vi "計算機.vi"() -> ()   [LabVIEW 2021]
uses:
  <vilib>/gmath/NI_Gmath.lvlib
  <vilib>/regexp/Match Regular Expression.xnode
panel:
  out "113550059":string
  in  "+/-":bool
  in  "1/x":bool
  in  "stop":bool
  out "String 2":string
  in  "pi":bool
  in  "tan":bool
  in  "cos":bool
  in  "sin":bool
  in  "√":bool
  out "String":string
  out "concatenated string":string
  in  "%":bool
  in  "Del":bool
  in  "=":bool
  in  "CE":bool
  in  ")":bool
  in  "(":bool
  out "Answer":string
  in  "1":bool
  in  "/":bool
  in  ".":bool
  in  "0":bool
  in  "*":bool
  in  "3":bool
  in  "2":bool
  in  "-":bool
  in  "6":bool
  in  "5":bool
  in  "4":bool
  in  "+":bool
  in  "9":bool
  in  "8":bool
  in  "7":bool
  # "記錄一"
  # "記錄二"
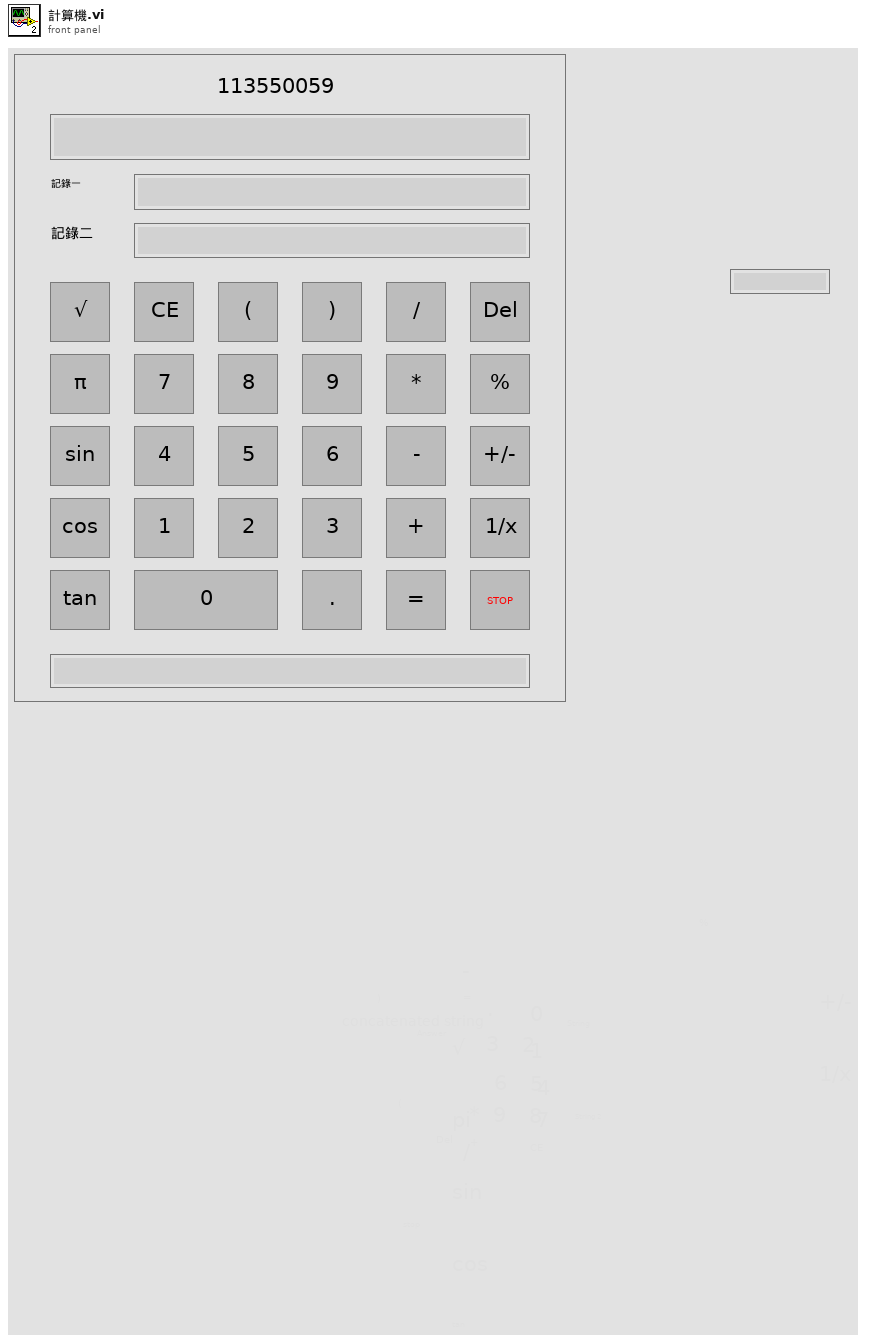
[diagram p1: front panel]
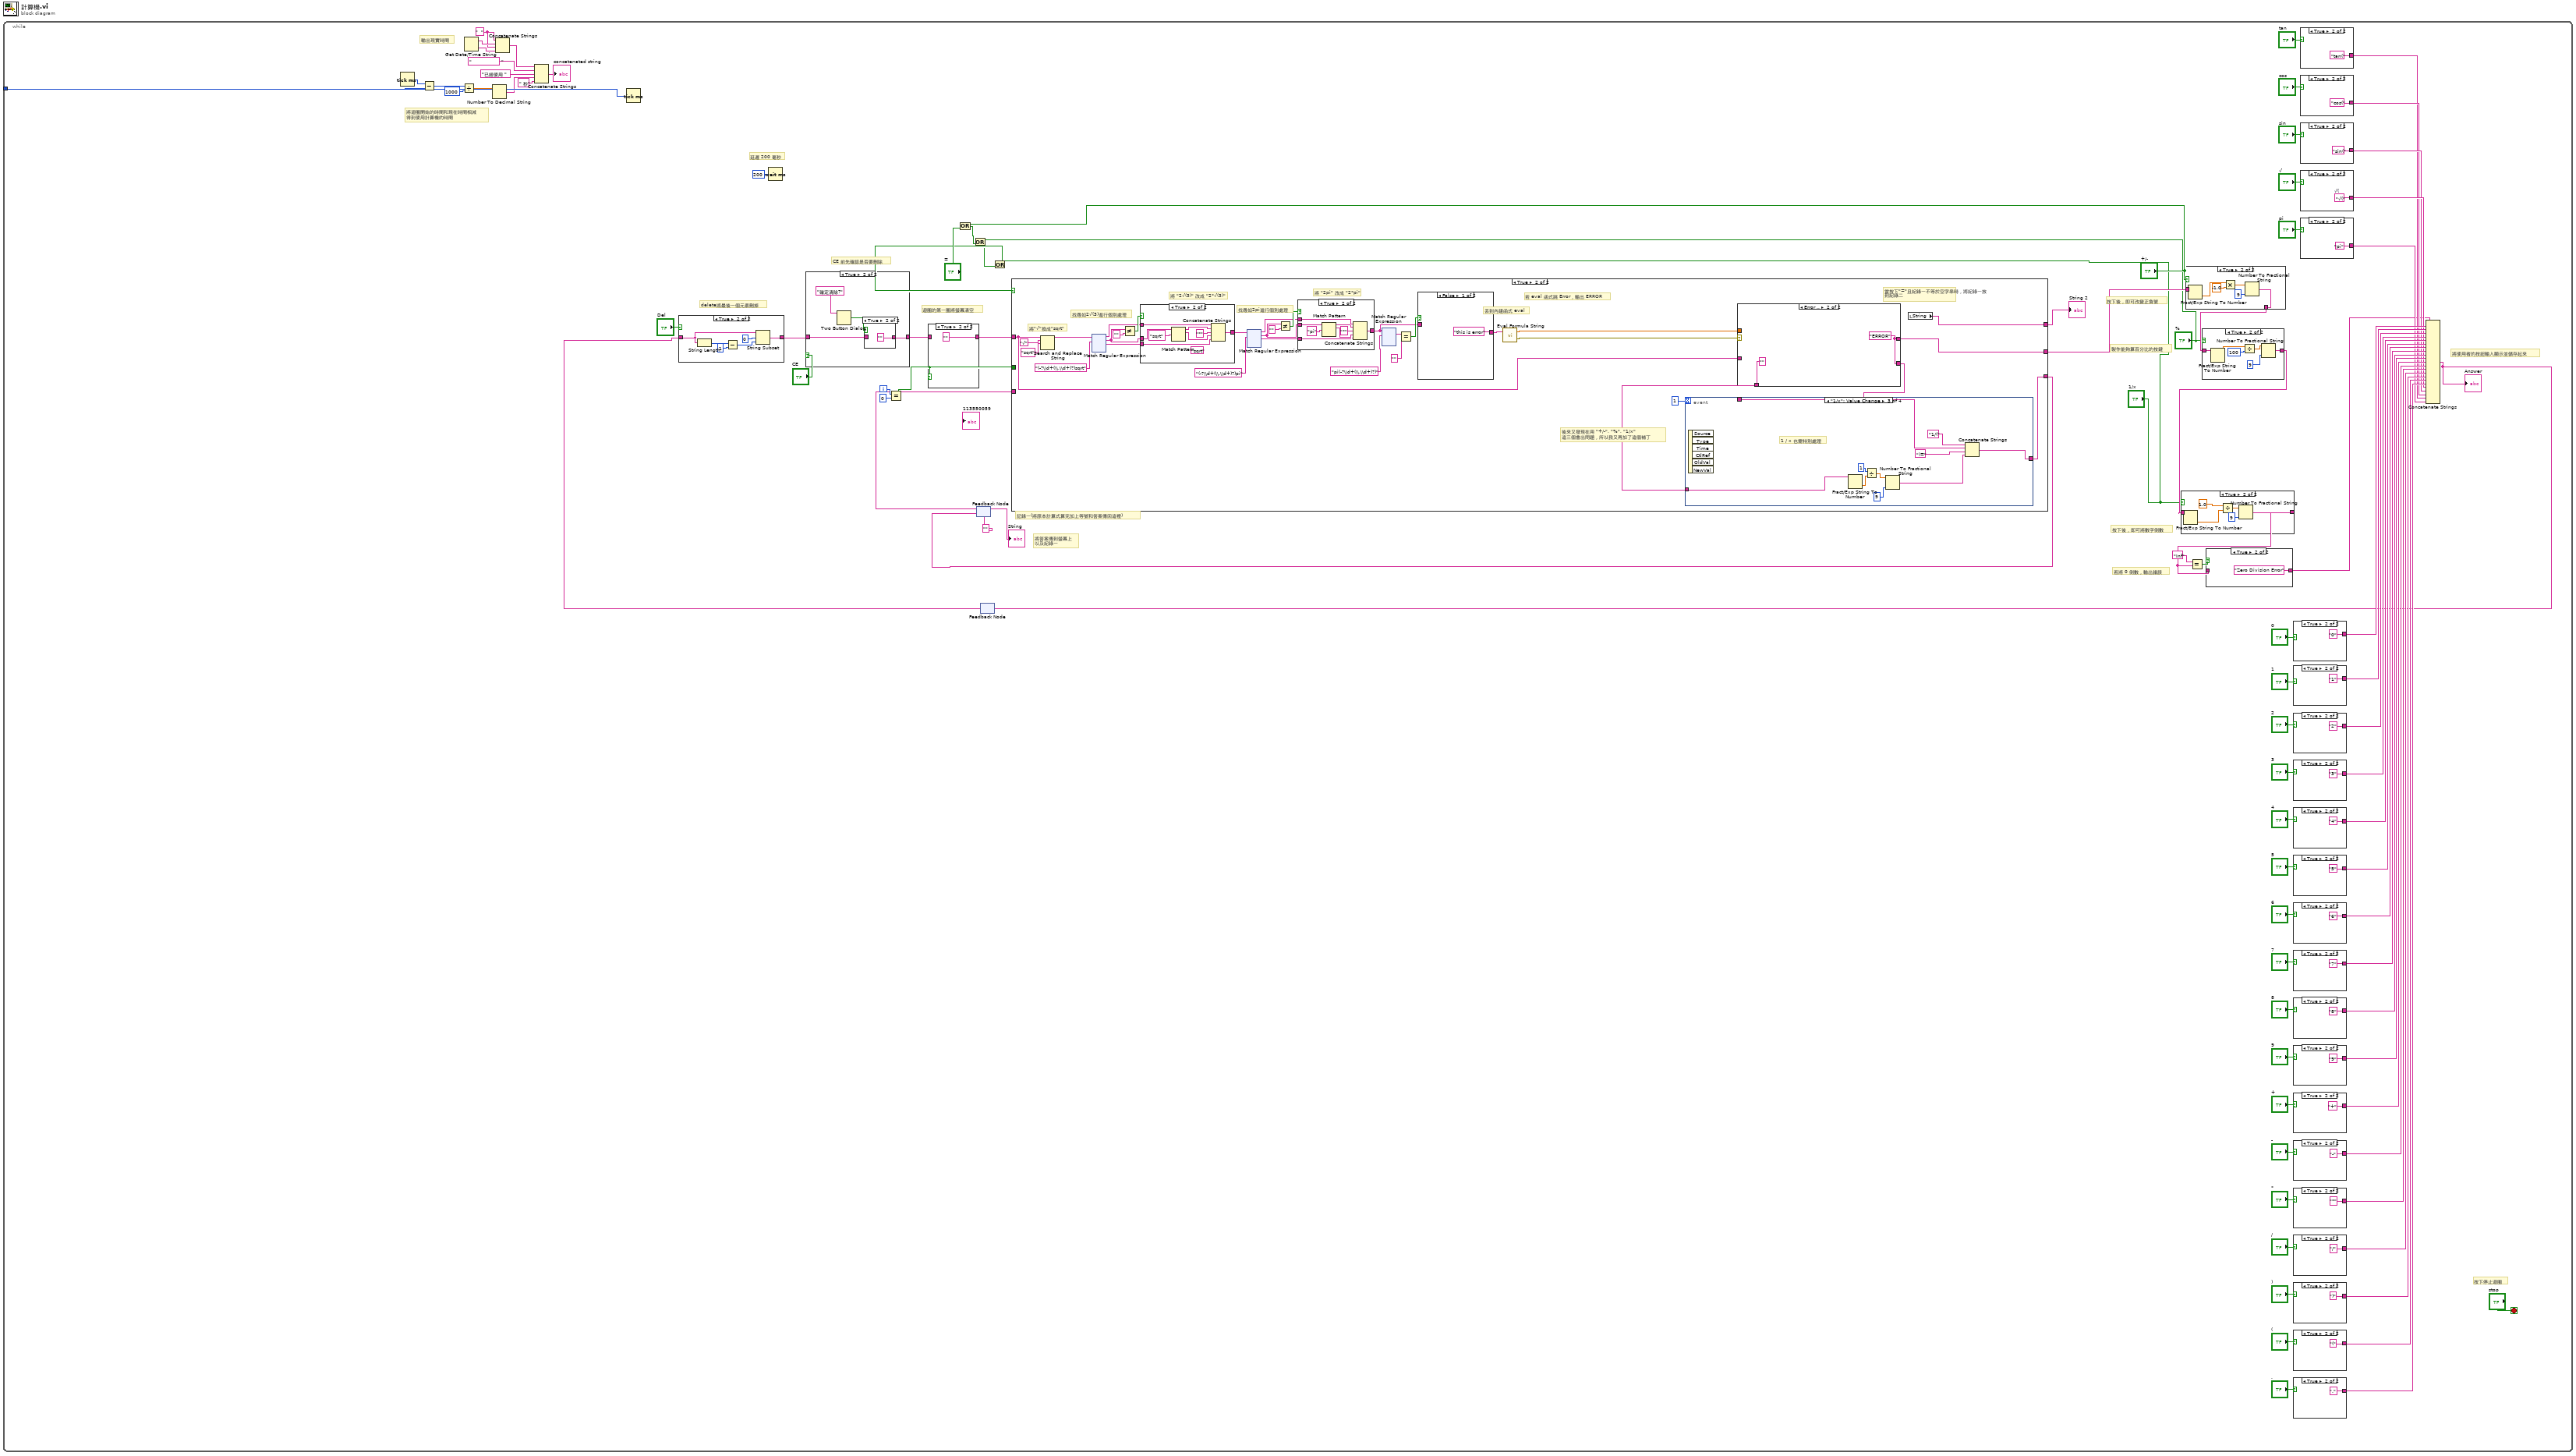
[diagram p0: block diagram]
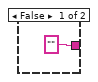
[diagram p7: hidden frame]
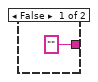
[diagram p8: hidden frame]
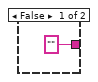
[diagram p9: hidden frame]
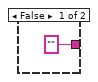
[diagram p10: hidden frame]
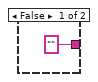
[diagram p11: hidden frame]
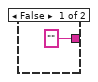
[diagram p15: hidden frame]
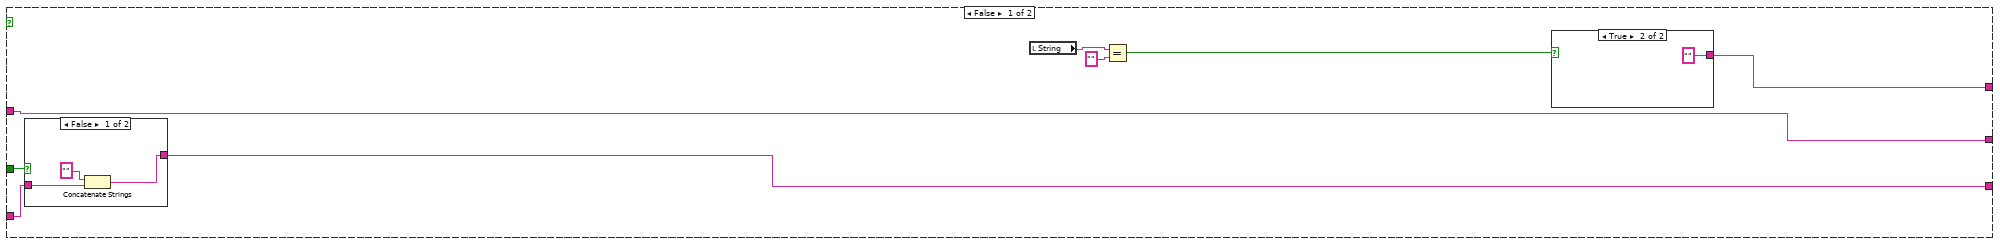
[diagram p16: hidden frame]
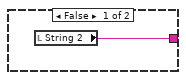
[diagram p17: hidden frame]
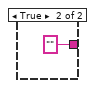
[diagram p18: hidden frame]
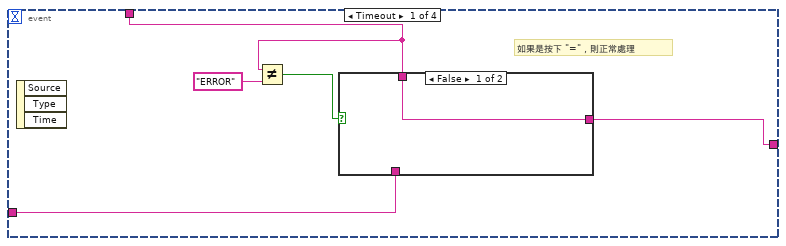
[diagram p19: hidden frame]
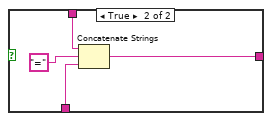
[diagram p20: hidden frame]
diagram:
  n1 = Tick Count (ms)() -> (millisecond timer value=w1:u32)
  n2 = while {
    tunnel: w1 -> [w29]
    i -> [w45]
    stop <- "stop" stop-if-true
    w24 = "  " ("string")
    # "按下後，即可改變正負號"
    # "若將 0 倒數，輸出錯誤"
    # "按下停止迴圈"
    # "延遲 200 毫秒"
    # "將答案傳到螢幕上\n以及紀錄一"
    # "迴圈的第一圈將螢幕清空"
    # "按下後，即可將數字倒數"
    # "delete將最後一個元素刪掉"
    # "輸出現實時間"
    # "將迴圈開始的時間和現在時間相減\n得到使用計算機的時間"
    # "製作能夠算百分比的按鍵"
    # "將使用者的按鈕輸入顯示並儲存起來"
    # "CE 前先確認是否要刪除"
    # "記錄一(將原本計算式算完加上等號和答案傳回這裡)"
    n3 = Tick Count (ms)() -> (millisecond timer value=w26:u32)
    n4 = Subtract(x=w26, y=w29) -> (x-y=w55:u32)
    n5 = Divide(x=w55, y=u32 1000) -> (x/y=w28:dbl)
    n6 = Get Date/Time String() -> (date string=w50:string, time string=w25:string)  [unwired: 3 in]
    n7 = Number To Decimal String(number=w28) -> (decimal integer string=w30:string)  [unwired: 1 in]
    n8 = Concatenate Strings(w24, w50, w24, w25) -> (w49:string)
    n9 = Concatenate Strings(w49, "                   ", "已經使用 ", w30, " 秒") -> (→"concatenated string":string)
    n10 = Wait (ms)(milliseconds to wait=u32 200) -> ()  [unwired: 1 out]
    n11 = Equal?(x=w45, y=0) -> (x = y?=w23:bool)
    n12 = Or(x="+/-", y="=") -> (x .or. y?=w12:bool)
    n13 = Or(x="%", y=w12) -> (x .or. y?=w4:bool)
    n14 = feedback #1("") -> (w33:string)
    "String" <- w33
    n15 = feedback #2() -> (w8:string)  [unwired: 1 in]
    n16 = case shown="True" "Del" {
      tunnel: w8 -> [w125 w131]
      tunnel: [w125 w126] -> w20
      frame False {
      }
      frame True {
        n17 = String Length(string=w131) -> (length=w129:i32)
        n18 = Subtract(x=w129, y=1) -> (x-y=w127:i32)
        n19 = String Subset(string=w131, offset (0)=0, length (rest)=w127) -> (substring=w126:string)
      }
    }
    n20 = case shown="True" "CE" {
      tunnel: w20 -> [w106 w108]
      tunnel: [w106 w107] -> w22
      frame False {
      }
      frame True {
        n21 = Two Button Dialog(message="確定清除?") -> (T button?=w110:bool)  [unwired: 2 in]
        n22 = case shown="True" w110 {
          tunnel: w108 -> [w111 _]
          tunnel: [w111 ""] -> w107
          frame False {
          }
          frame True {
          }
        }
      }
    }
    n23 = case shown="True" w23 {
      tunnel: w22 -> [w123 _]
      tunnel: [w123 ""] -> w44
      frame False {
      }
      frame True {
      }
    }
    n24 = Or(x="1/x", y=w4) -> (x .or. y?=w5:bool)
    n25 = case shown="True" w5 {
      tunnel: w44 -> [w141 w174]
      tunnel: [w141 w179] -> w17
      tunnel: [w146 w156] -> w2
      tunnel: w33 -> [w147 _]
      tunnel: w23 -> [w148 _]
      tunnel: [w142 w173] -> w31
      frame False {
        n26 = case shown="False" w148 {
          tunnel: w147 -> [w153 _]
          tunnel: [w152 ""] -> w146
          frame False {
            n27 = Concatenate Strings("", w153) -> (w152:string)
          }
          frame True {
          }
        }
        n28 = local read "String"() -> (w145:string)
        n29 = Equal?(x=w145, y="") -> (x = y?=w144:bool)
        n30 = case shown="True" w144 {
          tunnel: [w149 ""] -> w142
          frame False {
            n31 = local read "String 2"() -> (w149:string)
          }
          frame True {
          }
        }
      }
      frame True {
        # "後來又發現在用 \"+/-\", \"%\", \"1/x\"\n這三個會出問題，所以我又再加了這個補丁"
        # "當按下\"=\"且紀錄一不等於空字串時，將紀錄一放到紀錄二"
        # "丟到內建函式 eval"
        # "若 eval 函式跳 Error，輸出 ERROR"
        # "將 \"2pi\" 改成 \"2*pi\""
        # "找尋如2pi進行個別處理"
        # "將 \"2√(3)\" 改成 \"2*√(3)\""
        # "找尋如2√(3)進行個別處理"
        # "將\"√\"換成\"sqrt\""
        n32 = Search and Replace String(input string=w174, search string="√", replace string="sqrt") -> (result string=w165:string)  [unwired: 5 in, 3 out]
        n33 = xnode "Match Regular Expression"("input string"=w165, "regular expression"="(-?\\d+(\\.\\d+)?)sqrt") -> ("before match"=w169:string, "whole match"=w167:string, "after match"=w168:string)  [unwired: 4 in, 2 out]
        n34 = Not Equal?(x=w167, y="") -> (x != y?=w170:bool)
        n35 = case shown="True" w170 {
          tunnel: w169 -> [w378 w385]
          tunnel: w168 -> [w377 w380]
          tunnel: [w376 w381] -> w166
          tunnel: w167 -> [_ w379]
          frame False {
            n36 = Concatenate Strings(w378, w377) -> (w376:string)
          }
          frame True {
            (unwired) "sqrt"
            n37 = Match Pattern(string=w379, regular expression="sqrt") -> (before substring=w384:string, match substring=w382:string)  [unwired: 1 in, 2 out]
            n38 = Concatenate Strings(w385, w384, "*", w382, w380) -> (w381:string)
          }
        }
        n39 = xnode "Match Regular Expression"("input string"=w166, "regular expression"="(-?\\d+(\\.\\d+)?)pi") -> ("before match"=w182:string, "whole match"=w180:string, "after match"=w181:string)  [unwired: 4 in, 2 out]
        n40 = Not Equal?(x=w180, y="") -> (x != y?=w183:bool)
        n41 = case shown="True" w183 {
          tunnel: w182 -> [w519 w526]
          tunnel: w181 -> [w518 w521]
          tunnel: [w517 w522] -> w159
          tunnel: w180 -> [_ w520]
          frame False {
            n42 = Concatenate Strings(w519, w518) -> (w517:string)
          }
          frame True {
            n43 = Match Pattern(string=w520, regular expression="pi") -> (before substring=w525:string, match substring=w523:string)  [unwired: 1 in, 2 out]
            n44 = Concatenate Strings(w526, w525, "*", w523, w521) -> (w522:string)
          }
        }
        n45 = xnode "Match Regular Expression"("input string"=w159, "regular expression"="pi(-?\\d+(\\.\\d+)?)") -> ("whole match"=w162:string)  [unwired: 4 in, 4 out]
        n46 = Equal?(x=w162, y="") -> (x = y?=w160:bool)
        n47 = case shown="False" w160 {
          tunnel: ["this is error" w370] -> w163
          tunnel: w159 -> [_ w369]
          frame False {
          }
          frame True {
            # "將 pi 換成常數3.14.."
            n48 = Number To Fractional String(number=3.141592653589793, precision (6)=i16 15) -> (F-format string=w375:string)  [unwired: 2 in]
            n49 = Search and Replace String(replace all?=TRUE, input string=w369, search string="pi", replace string=w375) -> (result string=w370:string)  [unwired: 4 in, 3 out]
          }
        }
        n50 = call <vilib>:"Eval Formula String.vi"("formula"=w163) -> ("error out"=w177:errorcluster, "y value"=w178:dbl)  [unwired: 1 in]
        n51 = case shown="Error .." w177 {
          tunnel: w174 -> [w505 _]
          tunnel: [w506 w516] -> w157
          tunnel: [w509 w516] -> w179
          tunnel: w178 -> [w510 _]
          tunnel: [w504 ""] -> w155
          frame No Error {
            # "如果有INF，應為 /0 的問題"
            n52 = Number To Fractional String(number=w510, precision (6)=9) -> (F-format string=w504:string)  [unwired: 2 in]
            n53 = Equal?(x=w504, y="Inf") -> (x = y?=w507:bool)
            n54 = case shown="True" w507 {
              tunnel: w504 -> [w513 _]
              tunnel: [w513 w514] -> w509
              tunnel: w505 -> [w512 _]
              tunnel: [w512 w514] -> w506
              frame False {
              }
              frame True {
                w514 = "Zero Division Error"
              }
            }
          }
          frame Error {
            w516 = "ERROR"
          }
        }
        n55 = event shown="[2] \"1/x\": Value Change" {
          selector: _ -> [_ _ _ _]
          dyn-events: _ -> [_ _ _ _]
          timeout: 1 -> [_ _ _ _]
          tunnel: w157 -> [w188 w204 w212 w218]
          tunnel: [w189 w202 w211 w221] -> w156
          tunnel: w155 -> [w190 w198 w209 w220]
          event Timeout {
            # "如果是按下 \"=\"，則正常處理"
            n56 = event-data() -> ()  [unwired: 1 in, 3 out]
            n57 = Not Equal?(x=w188, y="ERROR") -> (x != y?=w186:bool)
            n58 = case shown="False" w186 {
              tunnel: w188 -> [w191 w195]
              tunnel: w190 -> [_ w194]
              tunnel: [w191 w193] -> w189
              frame False {
              }
              frame True {
                n59 = Concatenate Strings(w195, "=", w194) -> (w193:string)
              }
            }
          }
          event "%": Value Change {
            # "% 也需特別處理"
            n60 = event-data() -> ()  [unwired: 1 in, 6 out]
            n61 = Fract/Exp String To Number(string=w198) -> (number=w196:dbl)  [unwired: 3 in, 1 out]
            n62 = Divide(x=w196, y=100) -> (x/y=w199:dbl)
            n63 = Number To Fractional String(number=w199, precision (6)=9) -> (F-format string=w197:string)  [unwired: 2 in]
            n64 = Concatenate Strings(w204, "%=", w197) -> (w202:string)
          }
          event "1/x": Value Change {
            # "1 / x 也需特別處理"
            n65 = event-data() -> ()  [unwired: 1 in, 6 out]
            n66 = Fract/Exp String To Number(string=w209) -> (number=w207:dbl)  [unwired: 3 in, 1 out]
            n67 = Divide(x=1, y=w207) -> (x/y=w206:dbl)
            n68 = Number To Fractional String(number=w206, precision (6)=9) -> (F-format string=w205:string)  [unwired: 2 in]
            n69 = Concatenate Strings("1/(", w212, ")=", w205) -> (w211:string)
          }
          event "+/-": Value Change {
            n70 = event-data() -> ()  [unwired: 1 in, 5 out]
            n71 = Equal?(x=w218, y="-0.000000000") -> (x = y?=w216:bool)
            n72 = Equal?(x=w218, y="0.000000000") -> (x = y?=w217:bool)
            n73 = Or(x=w217, y=w216) -> (x .or. y?=w215:bool)
            n74 = case shown="False" w215 {
              tunnel: w218 -> [w225 _]
              tunnel: [w224 "0.000000000=0.00000000"] -> w221
              tunnel: w220 -> [w223 _]
              frame False {
                # "按下 \"+/-\"，則判斷是正是負或是 0 來處理"
                n75 = Fract/Exp String To Number(string=w223) -> (number=w233:dbl)  [unwired: 3 in, 1 out]
                n76 = String Subset(string=w225, offset (0)=0, length (rest)=1) -> (substring=w231:string)
                n77 = Multiply(x=-1, y=w233) -> (x*y=w234:dbl)
                n78 = Equal?(x=w231, y="-") -> (x = y?=w232:bool)
                n79 = Number To Fractional String(number=w234, precision (6)=9) -> (F-format string=w235:string)  [unwired: 2 in]
                n80 = case shown="True" w232 {
                  tunnel: w225 -> [w241 w248]
                  tunnel: [w236 w242] -> w224
                  tunnel: w235 -> [w237 w244]
                  frame False {
                    n81 = Concatenate Strings("-", w241) -> (w238:string)
                    n82 = Concatenate Strings(w238, "=", w237) -> (w236:string)
                  }
                  frame True {
                    n83 = String Length(string=w248) -> (length=w246:i32)
                    n84 = Decrement(x=w246) -> (x-1=w247:i32)
                    n85 = String Subset(string=w248, offset (0)=1, length (rest)=w247) -> (substring=w243:string)
                    n86 = Concatenate Strings(w243, "=", w244) -> (w242:string)
                  }
                }
              }
              frame True {
              }
            }
          }
        }
        n87 = local read "String"() -> (w173:string)
      }
    }
    "String 2" <- w31
    n88 = feedback-in #1(w2) -> ()
    n89 = case shown="True" "+/-" {
      tunnel: [w90 w95] -> w13
      tunnel: w17 -> [w90 w93]
      frame False {
      }
      frame True {
        n90 = Fract/Exp String To Number(string=w93) -> (number=w94:dbl)  [unwired: 3 in, 1 out]
        n91 = Multiply(x=w94, y=-1.0) -> (x*y=w96:dbl)
        n92 = Number To Fractional String(number=w96, precision (6)=i16 9) -> (F-format string=w95:string)  [unwired: 2 in]
      }
    }
    n93 = case shown="True" "%" {
      tunnel: w13 -> [w132 w137]
      tunnel: [w132 w138] -> w7
      frame False {
      }
      frame True {
        n94 = Fract/Exp String To Number(string=w137) -> (number=w136:dbl)  [unwired: 3 in, 1 out]
        n95 = Divide(x=w136, y=100) -> (x/y=w134:dbl)
        n96 = Number To Fractional String(number=w134, precision (6)=9) -> (F-format string=w138:string)  [unwired: 2 in]
      }
    }
    n97 = case shown="True" "1/x" {
      tunnel: [w99 w105] -> w10
      tunnel: w7 -> [w99 w104]
      frame False {
      }
      frame True {
        n98 = Fract/Exp String To Number(string=w104) -> (number=w101:dbl)  [unwired: 3 in, 1 out]
        n99 = Divide(x=1.0, y=w101) -> (x/y=w100:dbl)
        n100 = Number To Fractional String(number=w100, precision (6)=i16 9) -> (F-format string=w105:string)  [unwired: 2 in]
      }
    }
    n101 = Equal?(x="Inf", y=w10) -> (x = y?=w18:bool)
    n102 = case shown="True" w18 {
      tunnel: w10 -> [w97 _]
      tunnel: [w97 "Zero Division Error"] -> w6
      frame False {
      }
      frame True {
      }
    }
    n103 = case shown="True" "0" {
      tunnel: ["" "0"] -> w88
      frame False {
      }
      frame True {
      }
    }
    n104 = case shown="True" "1" {
      tunnel: ["" "1"] -> w86
      frame False {
      }
      frame True {
      }
    }
    n105 = case shown="True" "2" {
      tunnel: ["" "2"] -> w77
      frame False {
      }
      frame True {
      }
    }
    n106 = case shown="True" "3" {
      tunnel: ["" "3"] -> w76
      frame False {
      }
      frame True {
      }
    }
    n107 = case shown="True" "4" {
      tunnel: ["" "4"] -> w75
      frame False {
      }
      frame True {
      }
    }
    n108 = case shown="True" "5" {
      tunnel: ["" "5"] -> w74
      frame False {
      }
      frame True {
      }
    }
    n109 = case shown="True" "6" {
      tunnel: ["" "6"] -> w73
      frame False {
      }
      frame True {
      }
    }
    n110 = case shown="True" "7" {
      tunnel: ["" "7"] -> w72
      frame False {
      }
      frame True {
      }
    }
    n111 = case shown="True" "8" {
      tunnel: ["" "8"] -> w71
      frame False {
      }
      frame True {
      }
    }
    n112 = case shown="True" "9" {
      tunnel: ["" "9"] -> w70
      frame False {
      }
      frame True {
      }
    }
    n113 = case shown="True" "+" {
      tunnel: ["" "+"] -> w63
      frame False {
      }
      frame True {
      }
    }
    n114 = case shown="True" "-" {
      tunnel: ["" "-"] -> w62
      frame False {
      }
      frame True {
      }
    }
    n115 = case shown="True" "*" {
      tunnel: ["" "*"] -> w61
      frame False {
      }
      frame True {
      }
    }
    n116 = case shown="True" "/" {
      tunnel: ["" "/"] -> w60
      frame False {
      }
      frame True {
      }
    }
    n117 = case shown="True" ")" {
      tunnel: ["" ")"] -> w59
      frame False {
      }
      frame True {
      }
    }
    n118 = case shown="True" "(" {
      tunnel: ["" "("] -> w58
      frame False {
      }
      frame True {
      }
    }
    n119 = case shown="True" "." {
      tunnel: ["" "."] -> w56
      frame False {
      }
      frame True {
      }
    }
    n120 = case shown="True" "tan" {
      tunnel: ["" "tan("] -> w36
      frame False {
      }
      frame True {
      }
    }
    n121 = case shown="True" "cos" {
      tunnel: ["" "cos("] -> w37
      frame False {
      }
      frame True {
      }
    }
    n122 = case shown="True" "sin" {
      tunnel: ["" "sin("] -> w38
      frame False {
      }
      frame True {
      }
    }
    n123 = case shown="True" "√" {
      tunnel: ["" w122] -> w42
      frame False {
      }
      frame True {
        w122 = "√("  # √(
      }
    }
    n124 = case shown="True" "pi" {
      tunnel: ["" "pi"] -> w34
      frame False {
      }
      frame True {
      }
    }
    n125 = Concatenate Strings(w6, w88, w86, w77, w76, w75, w74, w73, w72, w71, w70, w63, w62, w61, w60, w59, w58, w56, w42, w38, w37, w36, w34) -> (w14:string)
    "Answer" <- w14
    n126 = feedback-in #2(w14) -> ()
  }
